vi "Init Calibration.vi"(8 "error in (no error)":errorcluster, 11 "Red Pitaya Digitizer in":refnum<class "Red Pitaya Digitizer.lvclass">) -> (0 "error out":errorcluster, 3 "Red Pitaya Digitizer out":refnum<class "Red Pitaya Digitizer.lvclass">)   [LabVIEW 2021, in "Red Pitaya Digitizer.lvclass"]
uses:
  Red Pitaya Digitizer.lvclass
  Red Pitaya Digitizer.lvclass/Red Pitaya Digitizer.ctl
  6c2c9369-63ce-4712-8390-7e6283614e92.vi
  RP Core/RP Instrument/RP Instrument.lvclass
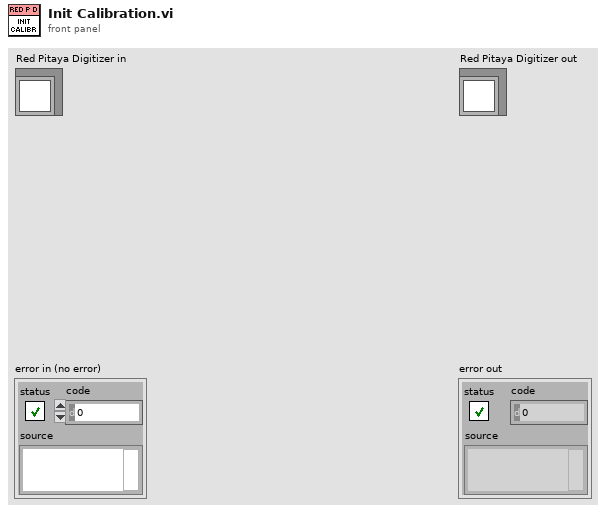
[diagram p1: front panel]
types:
  T1 = typedef "Lockin Digitizer Configuration.ctl" = cluster{"Post-trigger delay":dbl, "Post-trigger duration":dbl, "Rate":dbl, "Ranges":dbl[], "Re-name channels":string[], "Active channels":string, "External\nclock":bool, "Frequencies":dbl[], "Time\nconstant":dbl, "Output \namplitudes":dbl[], "Input\nchannles":string[]}
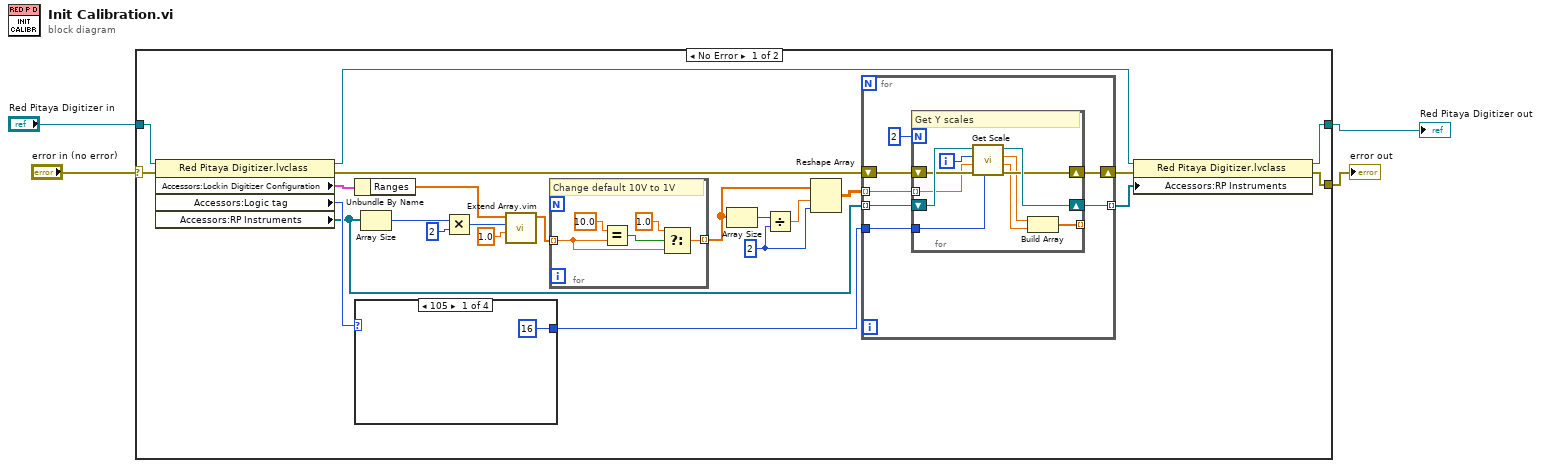
[diagram p0: block diagram]
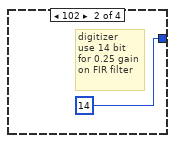
[diagram p2: hidden frame]
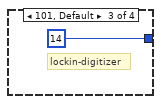
[diagram p3: hidden frame]
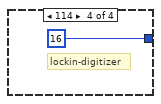
[diagram p4: hidden frame]
diagram:
  n1 = case shown="No Error" "error in (no error)" {
    selector: "error in (no error)" -> [w27 w55]
    tunnel: [w5 w55] -> w1
    tunnel: [w6 w54] -> w2
    tunnel: "Red Pitaya Digitizer in" -> [w26 w54]
    frame No Error {
      w8 = 2 ("dimension size")
      n2 = property class="Red Pitaya Digitizer.lvclass"(reference=w26, error in=w27) -> (reference out=w15:refnum<class "Red Pitaya Digitizer.lvclass">, error out=w13:errorcluster, "Accessors:Lockin Digitizer Configuration"=w25:T1, "Accessors:Logic tag"=w24:u16, "Accessors:RP Instruments"=w16:refnum<class "RP Instrument.lvclass">[])
      n3 = Unbundle By Name(w25) -> ("Ranges"=w20:dbl[])
      n4 = case shown="105" w24 {
        tunnel: [16 ("Signal bits") 14 ("Signal bits") 14 ("Signal bits") 16 ("Signal bits")] -> w23
        frame 105 {
        }
        frame 102 {
          # "digitizer\nuse 14 bit \nfor 0.25 gain\non FIR filter"
        }
        frame 101, Default {
          # "lockin-digitizer"
        }
        frame 114 {
          # "lockin-digitizer"
        }
      }
      n5 = Array Size(array=w16) -> (size(s)=w22:i32)
      n6 = Multiply(x=w22, y=2) -> (x*y=w18:i32)
      n7 = call "Extend Array.vim"("Default value"=1.0, "Extend to size"=w18, "Array in"=w20) -> ("Array out"=w17:dbl[])  [unwired: 7 in, 1 out]
      n8 = for {
        tunnel: w17 -> [w47] mode=indexing
        tunnel: [w45] -> w9 mode=indexing
        # "Change default 10V to 1V"
        n9 = Equal?(x=10.0, y=w47) -> (x = y?=w48:bool)
        n10 = Select(t=1.0, s=w48, f=w47) -> (s? t:f=w45:dbl)
      }
      n11 = Array Size(array=w9) -> (size(s)=w10:i32)
      n12 = Divide(x=w10, y=w8) -> (x/y=w7:dbl)
      n13 = Reshape Array(w9, w7, w8) -> (w11:dbl[][])
      n14 = for {
        tunnel: w23 -> [w34]
        tunnel: w11 -> [w33] mode=indexing
        tunnel: w16 -> [w32] mode=indexing
        tunnel: [w31] -> w14 mode=indexing
        shift-right: [w29] -> w12
        shift-left: w13 -> [w30]
        n15 = for {
          N: 2 -> [_]
          tunnel: w33 -> [w36] mode=indexing
          tunnel: [w44] -> _ mode=indexing
          tunnel: w34 -> [w35]
          shift-right: [w42] -> w31
          shift-left: w32 -> [w43]
          shift-right: [w40] -> w29
          shift-left: w30 -> [w41]
          i -> [w37]
          # "Get Y scales"
          n16 = call-dynamic "Get Scale.vi"("Signal bits"=w35, "error in (no error)"=w41, "Range"=w36, "Channel"=w37, "RP Instrument in"=w43) -> ("error out"=w40:errorcluster, "slope"=w38:dbl, "y intersept"=w39:dbl, "RP Instrument out"=w42:refnum<class "RP Instrument.lvclass">)  [unwired: 2 in, 1 out]
          n17 = Build Array(w39, w38) -> (w44:dbl[])
        }
      }
      n18 = property class="Red Pitaya Digitizer.lvclass"(reference=w15, error in=w12, "Accessors:RP Instruments"=w14) -> (reference out=w6:refnum<class "Red Pitaya Digitizer.lvclass">, error out=w5:errorcluster)
    }
    frame Error {
    }
  }
  "error out" <- w1
  "Red Pitaya Digitizer out" <- w2
